vi "SUBVI_radon.vi"(7 "Refresco(s)":dbl=5.0 caption="Elapsed Time (s)", 8 "Error In":errorcluster) -> (0 "Error Out":errorcluster, 3 "Nuevo?":bool, 5 "Remote?":bool)   [LabVIEW 2013]
doc: "Illustrates how to create and write a configuration settings file.\n\nInstructions:\nEnter values in the controls on the front panel then click on the Run Arrow.\nTo read the file, run Read Configuration Settings File.vi located in the file\\config.llb."
uses:
  datosGraficaRadonNumeric.ctl
  ANAIS_GLOBALES.vi
panel:
  out "Radon":T1 {"Empty8" format="%.1f"; "Empty7" format="%.1f"; "Empty6" format="%.1f"; "Empty5" format="%.1f"; "Pressure" format="%.1f"; "Humidity" format="%.1f"; "Temperature" format="%.1f"; "Radon" format="%.1f"}
  out "SUM=0?":bool
  out "Errores acum S":i32 caption="Elapsed Time (s)"
  out "Errores acum W":i32 caption="Elapsed Time (s)"
  out "Web":string caption="asd"
  out "Idx":i32 caption="Elapsed Time (s)"
  in  "stop":bool
  out "readDate":string caption="asd"
  out "measDate":string caption="asd"
  in  "Refresh":bool
  # "Monitor de radon AlphaGuard"
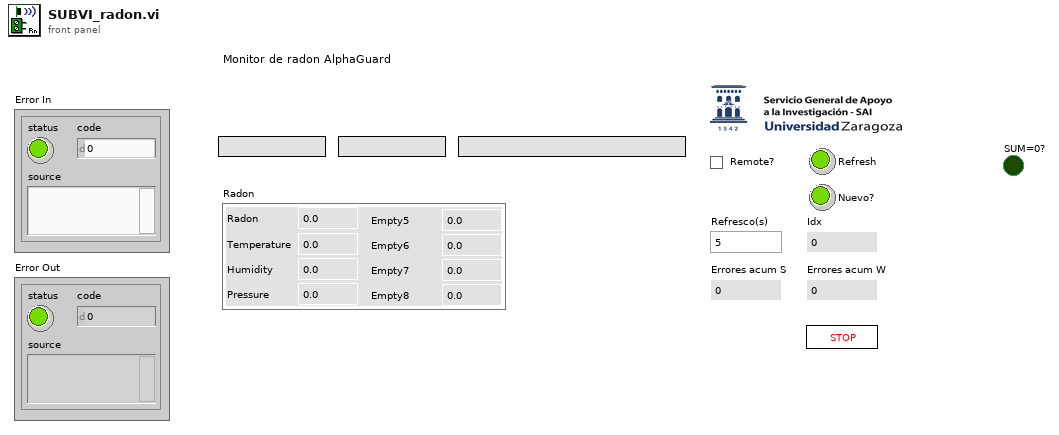
[diagram p1: front panel]
types:
  T1 = typedef "datosGraficaRadonNumeric.ctl" = cluster{"Radon":dbl, "Temperature":dbl, "Humidity":dbl, "Pressure":dbl, "Empty5":dbl, "Empty6":dbl, "Empty7":dbl, "Empty8":dbl}
  T2 = typedef "puertosIP.ctl" = cluster{"IMonWeb":string, "IMon":bool, "VMonWeb":string, "VMon":bool, "ClimatWeb":string, "Climat":bool, "RadonWeb":string, "Radon":bool, "BeagleEWeb":string, "BeagleE":bool, "BeagleDWeb":string, "BeagleD":bool, "RateWeb":string, "Rate":bool, "CratesWeb":string, "Crates":bool, "StartStopWeb":string, "StartStop":bool, "MuonRatesWeb":string, "MuonRates":bool, "N2LIQWeb":string, "N2LIQ":bool}
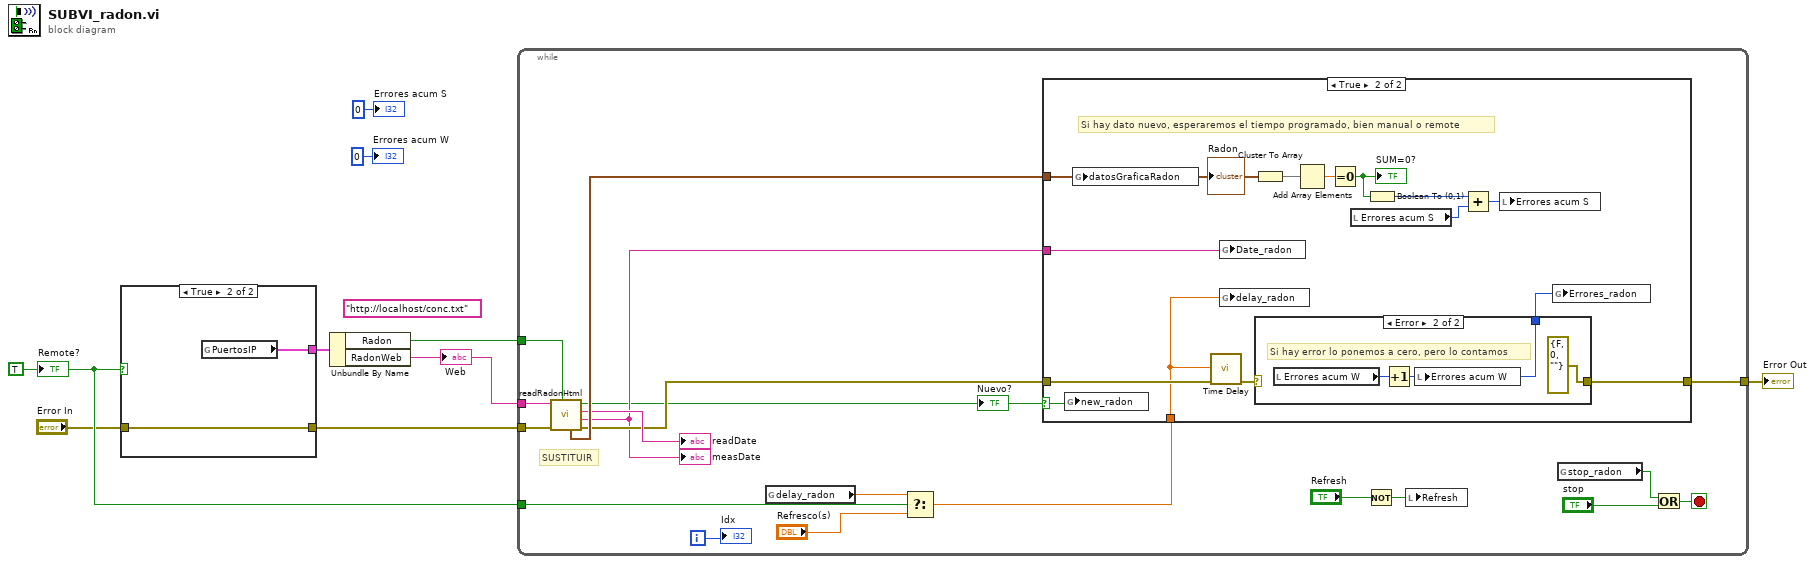
[diagram p0: block diagram]
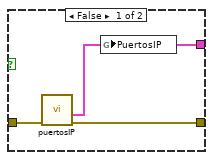
[diagram p2: hidden frame]
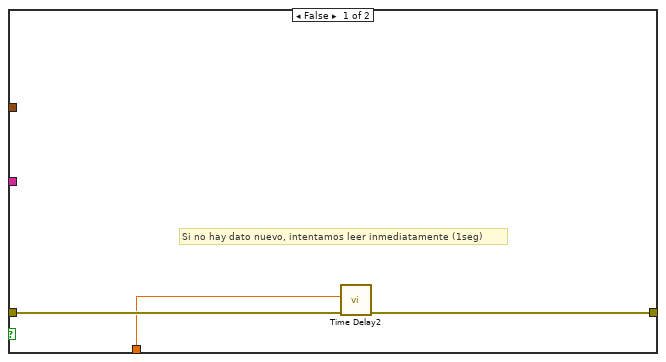
[diagram p3: hidden frame]
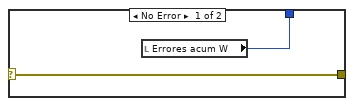
[diagram p4: hidden frame]
diagram:
  (unwired) "http://localhost/conc.txt" ("Web")
  w6 = TRUE ("Remote?")
  n1 = case shown="True" w6 {
    tunnel: [w12 w14] -> w8
    tunnel: "Error In" -> [w10 w13]
    tunnel: [w11 w13] -> w1
    frame False {
      n2 = call "puertosIP.vi"("error in (no error)"=w10) -> ("error out"=w11:errorcluster, "Cluster"=w12:T2)  [unwired: 8 in, 1 out]
      n3 = global write "ANAIS_GLOBALES.vi" "PuertosIP"(w12) -> ()
    }
    frame True {
      n4 = global read "ANAIS_GLOBALES.vi" "PuertosIP"() -> (w14:T2)
    }
  }
  n5 = Unbundle By Name(w8) -> ("Radon"=w4:bool, "RadonWeb"=w2:string)
  "Web" <- w2
  n6 = while {
    tunnel: [w20] -> w9
    tunnel: w6 -> [w25]
    tunnel: w2 -> [w24]
    tunnel: w1 -> [w23]
    tunnel: w4 -> [w17]
    i -> [w19]
    stop <- w30 stop-if-true
    # "SUSTITUIR"
    n7 = call "readRadonHtml.vi"("Web(T)"=w17, "Error In"=w23, "url"=w24) -> ("Error Out"=w18:errorcluster, "fechaMeas"=w16:string, "fechaRead"=→"readDate":string, "datoNuevo?"=w15:bool, "datosGraficaRadon"=w22:T1)  [unwired: 4 in]
    "measDate" <- w16
    "Nuevo?" <- w15
    n8 = global read "ANAIS_GLOBALES.vi" "delay_radon"() -> (w26:dbl)
    n9 = Select(t=w26, s=w25, f="Refresco(s)") -> (s? t:f=w27:dbl)
    n10 = case shown="True" w15 {
      selector: w15 -> [_ w37]
      tunnel: w27 -> [w34 w39]
      tunnel: w18 -> [w36 w50]
      tunnel: [w35 w48] -> w20
      tunnel: w22 -> [_ w38]
      tunnel: w16 -> [_ w40]
      frame False {
        # "Si no hay dato nuevo, intentamos leer inmediatamente (1seg)"
        n11 = call "Time Delay2"("error in (no error)"=w36, "Delay Time (s)"=w34) -> ("error out"=w35:errorcluster)  [unwired: 9 in]
      }
      frame True {
        # "Si hay dato nuevo, esperaremos el tiempo programado, bien manual o remote"
        n12 = global write "ANAIS_GLOBALES.vi" "new_radon"(w37) -> ()
        n13 = global write "ANAIS_GLOBALES.vi" "datosGraficaRadon"(w38) -> ()
        n14 = call "Time Delay"("error in (no error)"=w50, "Delay Time (s)"=w39) -> ("error out"=w49:errorcluster)  [unwired: 9 in]
        n15 = global write "ANAIS_GLOBALES.vi" "Date_radon"(w40) -> ()
        n16 = global write "ANAIS_GLOBALES.vi" "delay_radon"(w39) -> ()
        n17 = Cluster To Array(cluster=w38) -> (array=w45:dbl[])
        n18 = case shown="Error" w49 {
          selector: w49 -> [w51 _]
          tunnel: [w51 errorcluster {"status"=FALSE, "code"=0, "source"=""} ("error IO")] -> w48
          tunnel: [w52 w54] -> w41
          frame No Error {
            n19 = local read "Errores acum W"() -> (w52:i32)
          }
          frame Error {
            # "Si hay error lo ponemos a cero, pero lo contamos"
            n20 = local read "Errores acum W"() -> (w55:i32)
            n21 = Increment(x=w55) -> (x+1=w54:i32)
            n22 = local write "Errores acum W"(w54) -> ()
          }
        }
        n23 = Add Array Elements(numeric array=w45) -> (sum=w47:dbl)
        n24 = Equal To 0?(x=w47) -> (x = 0?=w43:bool)
        "SUM=0?" <- w43
        n25 = local read "Errores acum S"() -> (w46:i32)
        n26 = Boolean To (0,1)(Boolean=w43) -> (0, 1=w42:i16)
        n27 = Add(x=w42, y=w46) -> (x+y=w44:i32)
        n28 = local write "Errores acum S"(w44) -> ()
        n29 = global write "ANAIS_GLOBALES.vi" "Errores_radon"(w41) -> ()
        "Radon" <- w38
      }
    }
    n30 = Not(x="Refresh") -> (.not. x?=w31:bool)
    n31 = local write "Refresh"(w31) -> ()
    n32 = global read "ANAIS_GLOBALES.vi" "stop_radon"() -> (w29:bool)
    n33 = Or(x=w29, y="stop") -> (x .or. y?=w30:bool)
    "Idx" <- w19
  }
  "Error Out" <- w9
  "Remote?" <- w6
  "Errores acum W" <- 0 ("Errores acum.")
  "Errores acum S" <- 0 ("Errores acum")
